vi "KeyenceCVX.Global.vi"() -> ()   [LabVIEW 2016]
uses:
  KeyenceCVX.Data.Status.ctl
  KeyenceCVX.Data.Status.State.ctl
  private/controls/TriggerNo.ctl
  private/controls/RunMode.ctl
  KeyenceCVX.Data.Sets.ctl
  KeyenceCVX.CodeDetails.ctl
panel:
  out "KeyenceCVX.Stop":bool
  out "KeyenceCVX.ReadOut Details":T1
  in  "KeyenceCVX.Sets":T2
  out "KeyenceCVX.Status":T3 {"TriggerNo" items=["1"=1, "2"=2, "3"=3, "4"=4, "ALL"=5]}
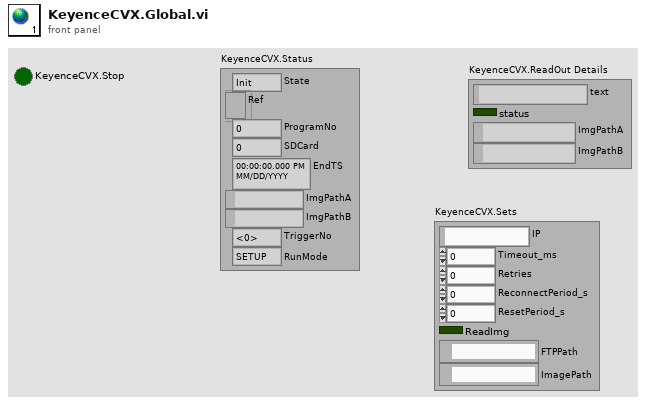
[diagram p1: front panel]
types:
  T1 = typedef "KeyenceCVX.CodeDetails.ctl" = cluster{"text":string, "status":bool, "ImgPathA":path, "ImgPathB":path}
  T2 = typedef "KeyenceCVX.Data.Sets.ctl" = cluster{"IP":string, "Timeout_ms":i32, "Retries":i32, "ReconnectPeriod_s":i32, "ResetPeriod_s":i32, "ReadImg":bool, "FTPPath":path, "ImagePath":path}
  T3 = typedef "KeyenceCVX.Data.Status.ctl" = cluster{"State":T4, "Ref":refnum<k5>, "ProgramNo":u16, "SDCard":u8, "EndTS":timestamp, "ImgPathA":path, "ImgPathB":path, "TriggerNo":T5, "RunMode":T6}
  T4 = typedef "KeyenceCVX.Data.Status.State.ctl" = enum16{"Init", "Idle", "Scan", "Reset", "ScanAck", "ChangeProgram"}
  T5 = typedef "TriggerNo.ctl" = u8
  T6 = typedef "RunMode.ctl" = enum16{"SETUP", "RUN"}
diagram:
